vi "from string.vi"(8 "error in":errorcluster, 9 "data":string, 10 "version":string, 11 "user tag bus module configuration In":refnum<class "user tag bus module configuration.lvclass">) -> (0 "error out":errorcluster, 3 "user tag bus module configuration Out":refnum<class "user tag bus module configuration.lvclass">)   [LabVIEW 2013, in "user tag bus module configuration.lvclass"]
doc: "Provides an interface for loading a module configuration from a file or other serialized data source. It is recommended that all children of this class store data in two sets--data required for its own initialization, and any data required for parent initialization--and that each implementation uses the <b>Call Parent Method</b> primitive to de-serialize parent information. As a result, it is expected that every module configuration class calls <b>component configuration.lvclass:From String.vi</b>."
uses:
  user tag bus module configuration.lvclass
  state module configuration.ctl
  <vilib>/NI/Tag Bus Module Framework/channel/TBM channel.lvclass
  <vilib>/NI/Tag Bus Module Framework/module configuration/TBM module configuration.lvclass
  user tag bus module configuration.lvclass/user tag bus module configuration.ctl
  <vilib>/NI/Tag Bus Module Framework/root configuration/TBM configuration.lvclass
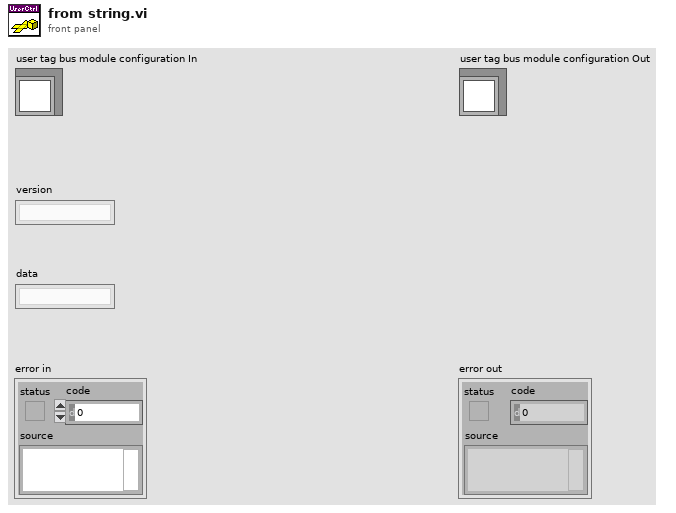
[diagram p1: front panel]
types:
  T1 = typedef "user tag bus module configuration.lvclass/state module configuration.ctl" = cluster{"fixed input":refnum<class "TBM channel.lvclass">, "fixed output":refnum<class "TBM channel.lvclass">, "initial state":u8}
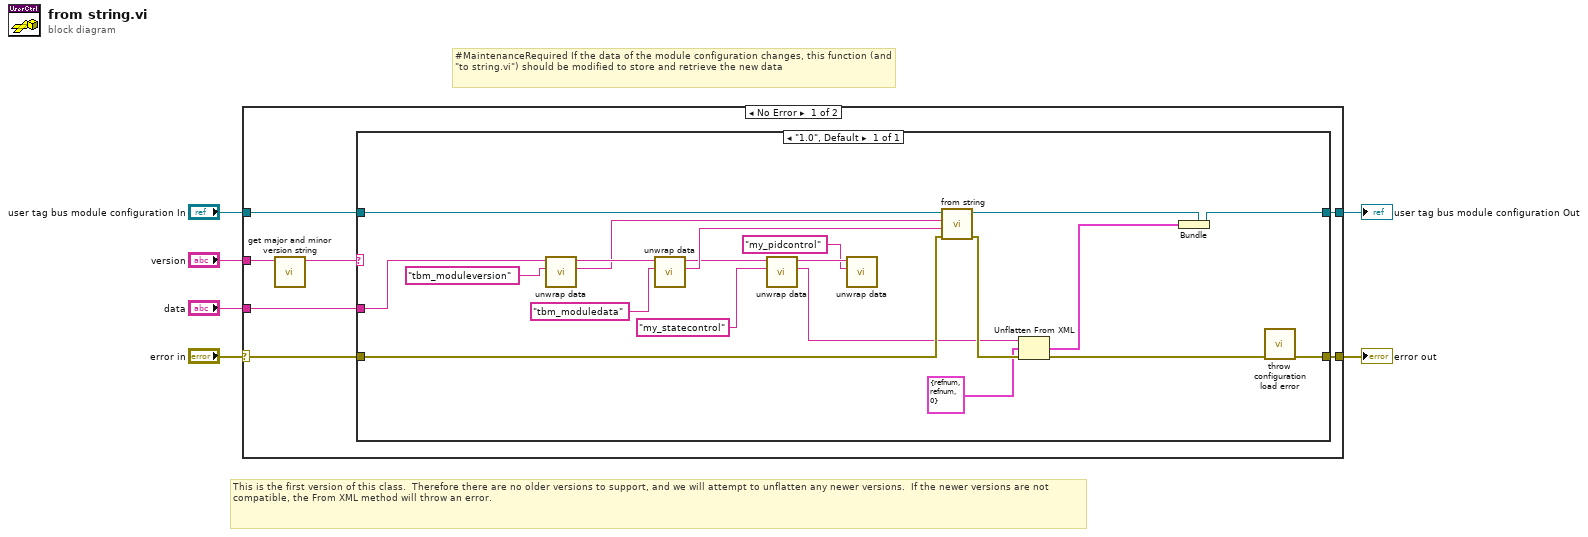
[diagram p0: block diagram]
diagram:
  # "#MaintenanceRequired If the data of the module configuration changes, this function (and \"to string.vi\") should be modified to store and retrieve the new data"
  # "This is the first version of this class.  Therefore there are no older versions to support, and we will attempt to unflatten any newer versions.  If the newer versions are not compatible, the From XML method will throw an error."
  n1 = case shown="No Error" "error in" {
    selector: "error in" -> [w7 w35]
    tunnel: "data" -> [w13 _]
    tunnel: "user tag bus module configuration In" -> [w12 w34]
    tunnel: [w11 w34] -> w5
    tunnel: [w10 w35] -> w4
    tunnel: "version" -> [w9 _]
    frame No Error {
      n2 = call <vilib>:"get major and minor version string.vi"("full version"=w9) -> ("major.minor version"=w8:string)  [unwired: 10 in]
      n3 = case shown="\"1.0\", Default" w8 {
        tunnel: w13 -> [w28]
        tunnel: w7 -> [w27]
        tunnel: w12 -> [w33]
        tunnel: [w22] -> w11
        tunnel: [w30] -> w10
        frame "1.0", Default {
          n4 = call <vilib>:"unwrap data.vi"("identifier"="tbm_moduleversion" ("additional identifier"), "data to unwrap"=w28) -> ("unwrapped data"=w23:string, "remaining string"=w29:string)  [unwired: 8 in]
          n5 = call <vilib>:"unwrap data.vi"("identifier"="tbm_moduledata" ("additional identifier"), "data to unwrap"=w29) -> ("unwrapped data"=w25:string, "remaining string"=w20:string)  [unwired: 8 in]
          n6 = call <vilib>:"unwrap data.vi"("identifier"="my_statecontrol" ("additional identifier"), "data to unwrap"=w20) -> ("unwrapped data"=w18:string, "remaining string"=w15:string)  [unwired: 8 in]
          n7 = call <vilib>:"unwrap data.vi"("identifier"="my_pidcontrol" ("additional identifier"), "data to unwrap"=w15) -> ()  [unwired: 8 in, 2 out]
          n8 = call-parent "from string.vi"("error in"=w27, "data"=w25, "version"=w23, "module configuration in"=w33) -> ("error out"=w31:errorcluster, "module configuration out"=w32:refnum<class "user tag bus module configuration.lvclass">)  [unwired: 6 in]
          n9 = Unflatten From XML(xml string=w18, type=T1 {"fixed input"=refnum, "fixed output"=refnum, "initial state"=0} ("state module configuration"), error in (no error)=w31) -> (value=w16:T1, error out=w21:errorcluster)
          n10 = Bundle(cluster=w32, w16) -> (w22:refnum<class "user tag bus module configuration.lvclass">)
          n11 = call <vilib>:"throw configuration load error.vi"("error in"=w21) -> ("error out"=w30:errorcluster)  [unwired: 10 in]
        }
      }
    }
    frame Error {
    }
  }
  "error out" <- w4
  "user tag bus module configuration Out" <- w5
